vi "Monitor Torque.vi"(0 "reference in":refnum<class "SmartMotor.lvclass">, 2 "Stop Motor Torque Monitor":bool, 4 "Max Monitoring Duration (ms)":u32=15000, 5 "error in (no error)":errorcluster) -> (14 "reference out":refnum<class "SmartMotor.lvclass">, 17 "Maxmum Torque":dbl, 18 "Screw Engaged":bool, 19 "error out":errorcluster)   [LabVIEW 2017, in "SmartMotor.lvclass"]
uses:
  SmartMotor.lvclass
  <vilib>/Analysis/baseanly.llb/Mean (DBL).vi
  <vilib>/Analysis/NI_AALBase.lvlib
panel:
  out "Passed Torque Limit":bool
  out "Waveform Chart":cluster{"Motor Torque":i32, "mean":dbl, dbl}(graph)
  # "NOTE: The Execution VI Properties for this VI must be set to reenterend.\n            When debugging set to default (non-reentrant)"
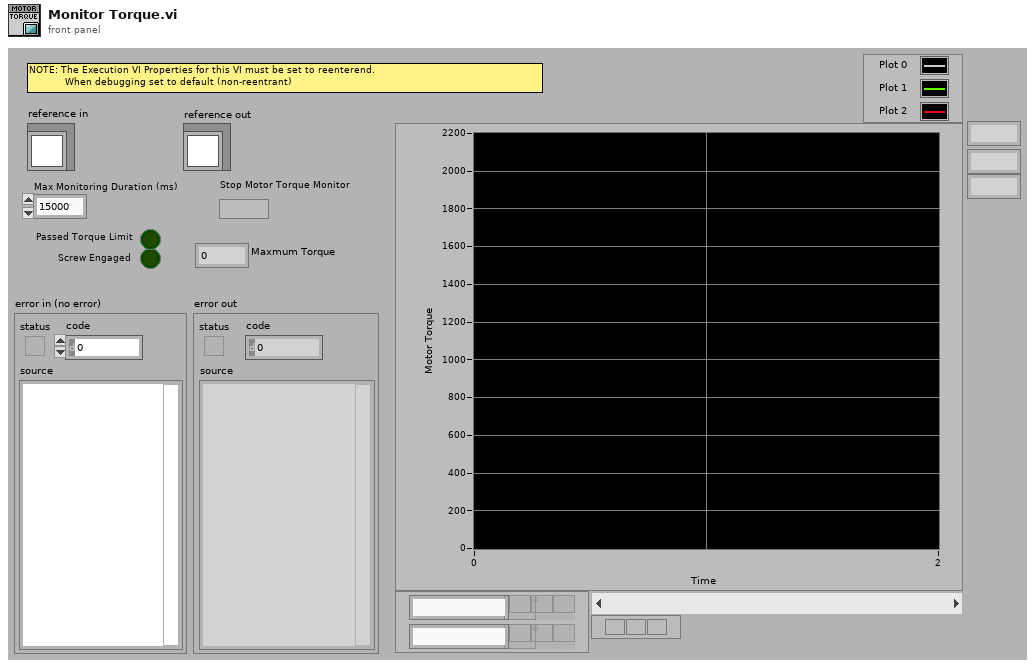
[diagram p1: front panel]
types:
  T1 = typedef "SmartMotor.lvclass/ObjectAttributes.ctl" = cluster{"SmartMotor Chain VISA Resource":refnum<visa-resource-name>, "SmartMotor Chain Address":i16, "Motor Absolute Position":i32, "Motor Relative Position":i32, "Motor Torque":i32, "Motor Voltage":i32, "Screwdriver Engaged":bool, "Screwdriver Torque Limit":i32, "Torque Monitor On/Off Status":bool, "Torque Monitor VI Reference":refnum<vi>, "Absolute Motor Torque (Filtered)":dbl, "SmartMotor Status":T2, "SmartMotor Error":T3}
  T2 = typedef "SmartMotor.lvclass/SmartMotor Status.ctl" = enum8{"Stopped", "Moving"}
  T3 = typedef "SmartMotor.lvclass/SmartMotor Error.ctl" = enum8{"None", "Read Error", "Low Voltage"}
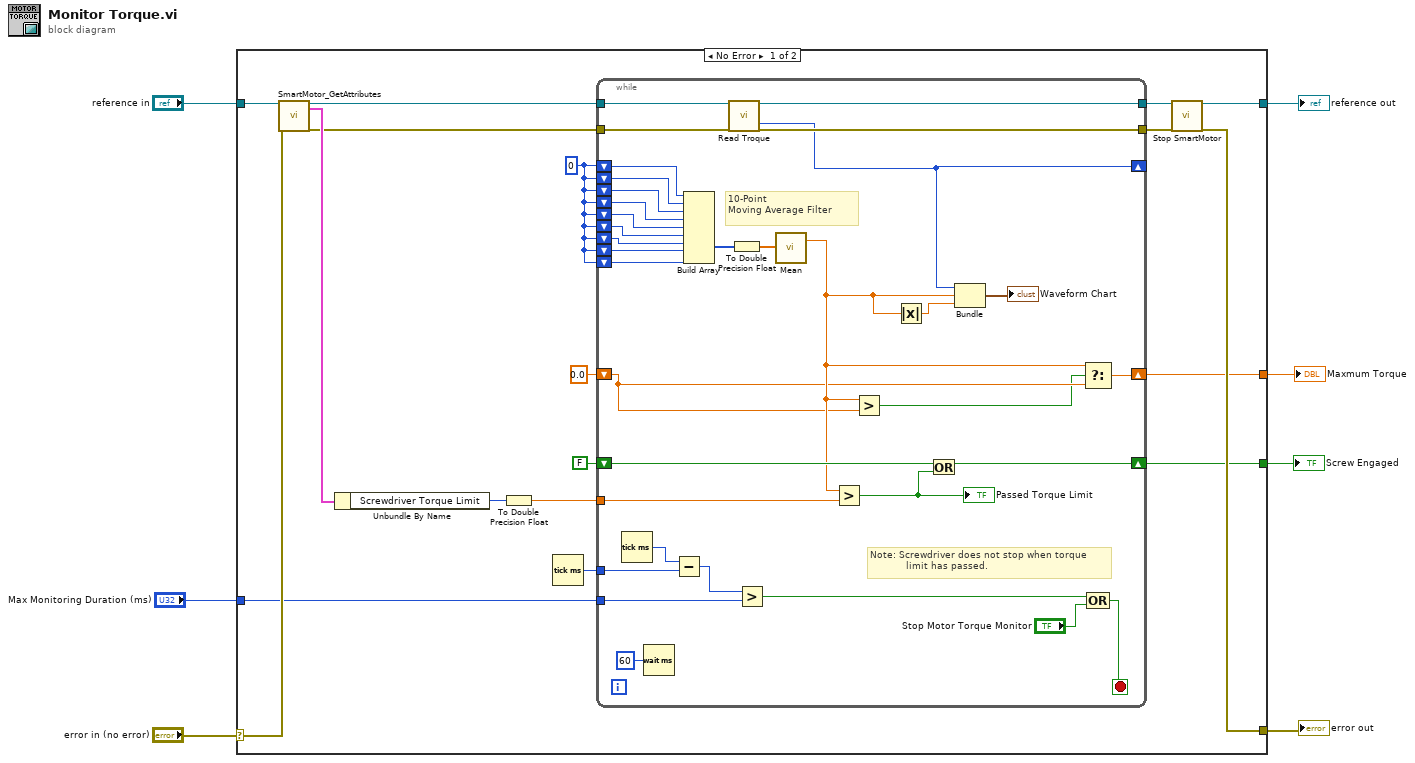
[diagram p0: block diagram]
diagram:
  n1 = case shown="No Error" "error in (no error)" {
    selector: "error in (no error)" -> [w24 w61]
    tunnel: [w17 w61] -> w6
    tunnel: [w10 w60] -> w4
    tunnel: "reference in" -> [w25 w60]
    tunnel: "Max Monitoring Duration (ms)" -> [w19 _]
    tunnel: [w13 _] -> w2
    tunnel: [w8 _] -> w1
    frame No Error {
      w11 = 0
      n2 = call "SmartMotor_GetAttributes.vi"("reference in"=w25, "error in (no error)"=w24) -> ("reference out"=w22:refnum<class "SmartMotor.lvclass">, "Data"=w23:T1, "error out"=w14:errorcluster)  [unwired: 14 in, 1 out]
      n3 = Unbundle By Name(w23) -> ("Screwdriver Torque Limit"=w18:i32)
      n4 = To Double Precision Float(number=w18) -> (double precision float=w21:dbl)
      n5 = Tick Count (ms)() -> (millisecond timer value=w20:u32)
      n6 = while {
        shift-right: [w32] -> _
        shift-left: w11 -> [w56]
        shift-left: w11 -> [w55]
        shift-left: w11 -> [w54]
        shift-left: w11 -> [w53]
        shift-left: w11 -> [w52]
        shift-left: w11 -> [w51]
        shift-left: w11 -> [w50]
        shift-left: w11 -> [w49]
        shift-left: w11 -> [w48]
        tunnel: [w39] -> w16
        tunnel: w22 -> [w43]
        tunnel: w21 -> [w42]
        tunnel: w20 -> [w41]
        tunnel: w19 -> [w40]
        tunnel: [w37] -> w15
        tunnel: w14 -> [w36]
        shift-right: [w33] -> w13
        shift-left: FALSE -> [w34]
        shift-right: [w29] -> w8
        shift-left: 0.0 ("mean") -> [w27]
        stop <- w38 stop-if-true
        # "Note: Screwdriver does not stop when torque\n            limit has passed."
        # "10-Point \nMoving Average Filter"
        n7 = Tick Count (ms)() -> (millisecond timer value=w46:u32)
        n8 = Wait (ms)(milliseconds to wait=u32 60) -> ()  [unwired: 1 out]
        n9 = Subtract(x=w46, y=w41) -> (x-y=w45:u32)
        n10 = Build Array(w56, w55, w54, w53, w52, w51, w50, w49, w48) -> (w57:i32[])
        n11 = call-dynamic "Read Troque.vi"("reference in"=w43, "error in (no error)"=w36) -> ("reference out"=w37:refnum<class "SmartMotor.lvclass">, "Motor Torque"=w32:i32, "error out"=w39:errorcluster)  [unwired: 15 in]
        n12 = To Double Precision Float(number=w57) -> (double precision float=w58:dbl[])
        n13 = Greater?(x=w45, y=w40) -> (0:w44:bool)
        n14 = call-poly <vilib>:"Mean.vi"("X"=w58) -> ("mean"=w28:dbl)  [unwired: 1 out]
        n15 = Greater?(x=w28, y=w42) -> (0:w30:bool)
        "Passed Torque Limit" <- w30
        n16 = Greater?(x=w28, y=w27) -> (0:w26:bool)
        n17 = Absolute Value(x=w28) -> (abs(x)=w31:dbl)
        n18 = Or(x=w34, y=w30) -> (x .or. y?=w33:bool)
        n19 = Bundle("Motor Torque"=w32, "mean"=w28, w31) -> (→"Waveform Chart":cluster{"Motor Torque":i32, "mean":dbl, dbl})  [unwired: 1 in]
        n20 = Select(t=w28, s=w26, f=w27) -> (s? t:f=w29:dbl)
        n21 = Compound Arithmetic op=OR(w44, "Stop Motor Torque Monitor") -> (w38:bool)
      }
      n22 = call-dynamic "Stop SmartMotor.vi"("reference in"=w15, "error in (no error)"=w16) -> ("reference out"=w10:refnum<class "SmartMotor.lvclass">, "error out"=w17:errorcluster)  [unwired: 16 in]
    }
    frame Error {
    }
  }
  "error out" <- w6
  "reference out" <- w4
  "Screw Engaged" <- w2
  "Maxmum Torque" <- w1
